vi "Result_Test.vi"(8 "error in (no error)":errorcluster caption="entrée d'erreur (pas d'erreur)", 11 "Delay en entrée":refnum<class "Enter_EMS_Code.lvclass">) -> (0 "error out":errorcluster caption="sortie d'erreur", 3 "Delay en sortie":refnum<class "Enter_EMS_Code.lvclass">)   [LabVIEW 2020, in "Library Test.lvlib" / "Enter_EMS_Code.lvclass"]
uses:
  Enter_EMS_Code.lvclass
  C:/Users/ngarcin/OneDrive - Altyor/Standard TB/Suite TB45/Class/Test/Test (Default)/Test (Default).lvclass
  Commun VI/TypeDef/Variable Printable.ctl
  Test_Without_Instr/Test_Without_Inst.lvclass
  Commun VI/Library Commun.lvlib
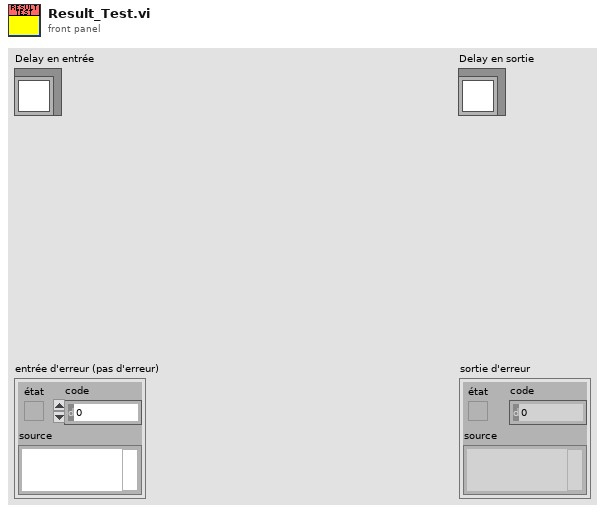
[diagram p1: front panel]
types:
  T1 = typedef "Variable Printable.ctl" = string
  T2 = enum16{"Get Variable", "Get All Variables", "Set Variable", "Delete Variable", "Delete All Variable"}
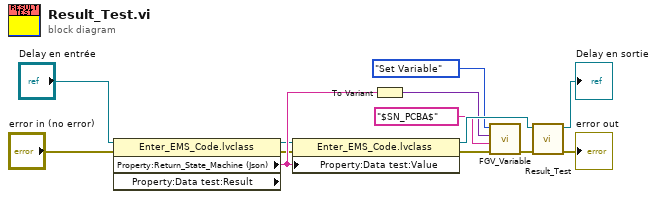
[diagram p0: block diagram]
diagram:
  n1 = property class="Enter_EMS_Code.lvclass" props=["Property:Return_State_Machine (Json)", "Property:Data test:Result"](reference="Delay en entrée", error in="error in (no error)") -> (reference out=w8:refnum<class "Enter_EMS_Code.lvclass">, error out=w6:errorcluster, "Property:Return_State_Machine (Json)"=w9:string)  [unwired: 1 out]
  n2 = property class="Enter_EMS_Code.lvclass"(reference=w8, error in=w6, "Property:Data test:Value"=w9) -> (reference out=w7:refnum<class "Enter_EMS_Code.lvclass">, error out=w1:errorcluster)
  n3 = To Variant(anything=w9) -> (Variant=w3:variant)
  n4 = call "FGV_Variable.vi"("error in (no error)"=w1, "Variable"=T1 "$SN_PCBA$", "Data In"=w3, "Function"=T2."Set Variable") -> ("error out"=w5:errorcluster)  [unwired: 5 in, 2 out]
  n5 = call-parent "Result_Test.vi"("error in (no error)"=w5, "Test_Without_Inst en entrée"=w7) -> ("error out"=→"error out":errorcluster, "Test_Without_Inst en sortie"=→"Delay en sortie":refnum<class "Enter_EMS_Code.lvclass">)  [unwired: 8 in]
